vi "rad_Deploy Image Wrapper_FB.vi"(4 "Deploy":string[](array[string]), 6 "restart after imaging (T)":bool=TRUE, 7 "Deployment Notifiers":T3, 8 "error in (no error)":errorcluster, 9 "apply primary NIC from image (F)":bool, 10 "image file path":path, 11 "Target settings in":T1={"Hostname"="", "Serial number"="", "Product name"="", "Product code"=0, "System status"="", "Credential type"=enum."None/Unlocked", "User added?"=FALSE, "Primary NIC"={"MAC address"="", "IP Address Request Mode"=2, "IP address"="", "Subnet mask"="", "Gateway"="", "DNS server"=""}} {"Primary NIC"."IP Address Request Mode" items=["Static"=1, "DHCP/Link-Local"=2, "Link-Local Only"=4, "DHCP Only"=8]}) -> (0 "error out":errorcluster, 2 "image file path":path, 3 "Target settings out":T1={"Hostname"="", "Serial number"="", "Product name"="", "Product code"=0, "System status"="", "Credential type"=enum."None/Unlocked", "User added?"=FALSE, "Primary NIC"={"MAC address"="", "IP Address Request Mode"=2, "IP address"="", "Subnet mask"="", "Gateway"="", "DNS server"=""}} {"Primary NIC"."IP Address Request Mode" items=["Static"=1, "DHCP/Link-Local"=2, "Link-Local Only"=4, "DHCP Only"=8]})   [LabVIEW 2016]
uses:
  TypeDefs/rad_Deployment Notifiers.ctl
  TypeDefs/rad_Deployment Status Data Type.ctl
  TypeDefs/rad_Deployment Progress Data Type.ctl
  Targets/TypeDefs/rad_Target Information.ctl
  Targets/TypeDefs/rad_Target Network Settings.ctl
  <vilib>/nisyscfg/Network Settings Image.ctl
  <vilib>/nisyscfg/Set System Image (Folder).vi
  <vilib>/nisyscfg/Close (System).vi
  <vilib>/nisyscfg/nisyscfg.lvlib
panel:
  out "Product name":string
  out "finished":bool
  in  "Stop Checking for Events":bool
  out "Progress":u8(slide) scale=0.0..100.0
  out "Status":string
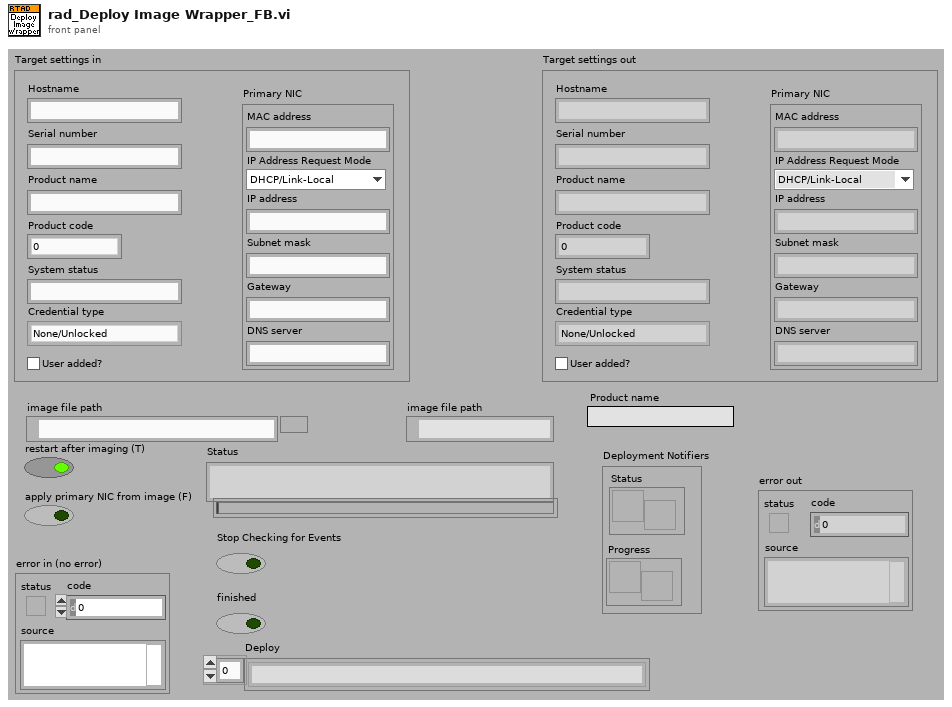
[diagram p1: front panel]
types:
  T1 = typedef "rad_Target Information.ctl" = cluster{"Hostname":string, "Serial number":string, "Product name":string, "Product code":i32, "System status":string, "Credential type":enum16{"None/Unlocked", "FTP Password", "NIAuth Credentials"}, "User added?":bool, "Primary NIC":T2}
  T2 = typedef "rad_Target Network Settings.ctl" = cluster{"MAC address":string, "IP Address Request Mode":i32, "IP address":string, "Subnet mask":string, "Gateway":string, "DNS server":string}
  T3 = typedef "rad_Deployment Notifiers.ctl" = cluster{"Status":refnum<notifier>, "Progress":refnum<notifier>}
  T4 = typedef "rad_Deployment Progress Data Type.ctl" = i8
  T5 = typedef "nisyscfg.lvlib/Network Settings Image.ctl" = u32
  T6 = enum32{"state changed", "beginning restart", "getting file", "putting file", "creating directory", "deleting file", "deleting directory", "enumerating file system", "renaming file", "current component", "operation progress", "downloading file", "unpacking file", "running install script"}
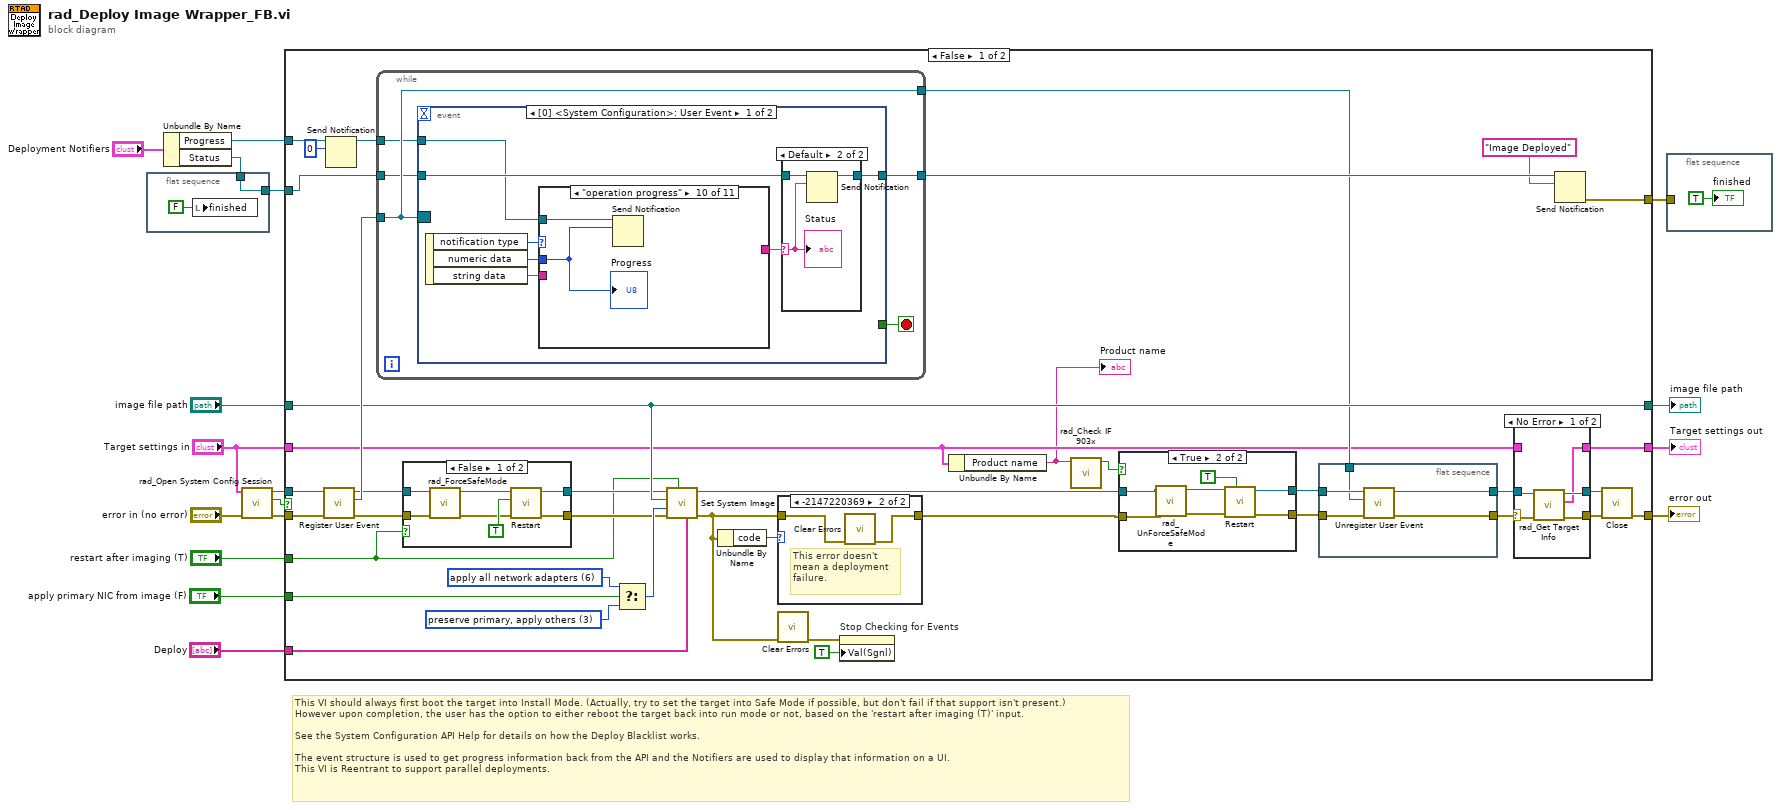
[diagram p0: block diagram]
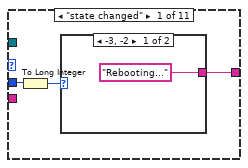
[diagram p7: hidden frame]
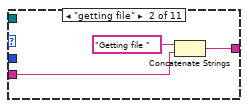
[diagram p9: hidden frame]
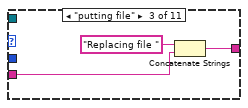
[diagram p10: hidden frame]
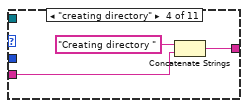
[diagram p11: hidden frame]
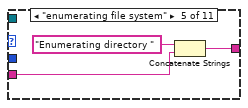
[diagram p12: hidden frame]
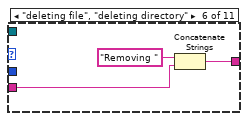
[diagram p13: hidden frame]
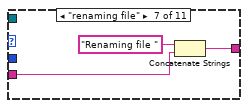
[diagram p14: hidden frame]
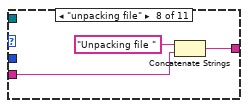
[diagram p15: hidden frame]
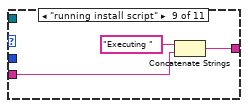
[diagram p16: hidden frame]
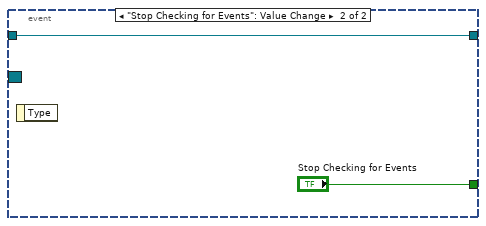
[diagram p18: hidden frame]
diagram:
  # "This VI should always first boot the target into Install Mode. (Actually, try to set the target into Safe Mode if possible, but don't fail if that support isn't present.)\nHowever upon completion, the user has the option to either reboot the target back into run mode or not, based on the 'restart after imaging (T)' input.\n\nSee the System Configuration API Help for details on how the Deploy Blacklist works.\n\nThe event structure is used to get progress information back from the API and the Notifiers are used to display that information on a UI. \nThis VI is Reentrant to support parallel deployments."
  n1 = flat-sequence {
    tunnel: [w18] -> w3
    tunnel: w2 -> [w18]
    frame #0 {
      n2 = local write "finished"(FALSE ("finished")) -> ()
    }
  }
  n3 = Unbundle By Name("Deployment Notifiers") -> ("Progress"=w11:refnum<notifier>, "Status"=w2:refnum<notifier>)
  n4 = call "rad_Open System Config Session.vi"("error in (no error)"="error in (no error)", "Target settings"="Target settings in") -> ("error out"=w7:errorcluster, "Cancelled"=w6:bool, "Session out"=w8:refnum<k21>)  [unwired: 6 in, 1 out]
  n5 = case shown="False" w6 {
    tunnel: [w58 w143] -> w17
    tunnel: "image file path" -> [w44 w142]
    tunnel: "restart after imaging (T)" -> [w37 _]
    tunnel: w8 -> [w57 _]
    tunnel: w7 -> [w56 w143]
    tunnel: [w52 _] -> w14
    tunnel: "apply primary NIC from image (F)" -> [w51 _]
    tunnel: w11 -> [w47 _]
    tunnel: [w44 w142] -> w16
    tunnel: "Deploy" -> [w43 _]
    tunnel: "Target settings in" -> [w26 w141]
    tunnel: [w34 w141] -> w4
    tunnel: w3 -> [w30 _]
    frame False {
      w50 = T5 6 items=["reset primary, disable others", "preserve primary, disable others", "preserve all network adapters", "preserve primary, apply others", "apply primary, disable others", "apply primary, preserve others", "apply all network adapters"] ("network settings (apply all adapters)")
      w49 = T5 3 items=["reset primary, disable others", "preserve primary, disable others", "preserve all network adapters", "preserve primary, apply others", "apply primary, disable others", "apply primary, preserve others", "apply all network adapters"] ("network settings (apply all adapters)")
      n6 = call <vilib>:"Register User Event.vi"("error in (no error)"=w56, "Session in"=w57) -> ("error out"=w40:errorcluster, "Event Registration out"=w55:refnum<event-registration>, "Session out"=w41:refnum<k21>)  [unwired: 7 in]
      n7 = Send Notification(notification=T4 0, notifier=w47) -> (notifier out=w46:refnum<notifier>)  [unwired: 1 in, 1 out]
      n8 = while {
        tunnel: w55 -> [w97]
        tunnel: [w97] -> w33
        tunnel: w30 -> [w95]
        tunnel: [w94] -> w54
        tunnel: w46 -> [w93]
        stop <- w96 stop-if-true
        n9 = event shown="[0] <System Configuration>: User Event" {
          selector: w97 -> [_ _]
          dyn-events: _ -> [_ _]
          timeout: _ -> [_ _]
          tunnel: [_ "Stop Checking for Events"] -> w96
          tunnel: w95 -> [w100 w139]
          tunnel: [w99 w139] -> w94
          tunnel: w93 -> [w98 _]
          event User Event {
            n10 = event-data() -> ("notification type"=w104:T6, "numeric data"=w102:u32, "string data"=w103:string)  [unwired: 1 in]
            n11 = case shown="\"operation progress\"" w104 {
              tunnel: [w109 w113 w116 w119 w122 w125 w128 w131 w134 _ _] -> w101
              tunnel: w103 -> [_ w114 w117 w120 w123 w126 w129 w132 w135 _ _]
              tunnel: w102 -> [w111 _ _ _ _ _ _ _ _ w138 _]
              tunnel: w98 -> [_ _ _ _ _ _ _ _ _ w137 _]
              frame "state changed" {
                n12 = To Long Integer(number=w111) -> (32bit integer=w110:i32)
                n13 = case shown="-3, -2" w110 {
                  tunnel: ["Rebooting..." _] -> w109
                  frame -3, -2 {
                  }
                  frame Default {
                  }
                }
              }
              frame "getting file" {
                n14 = Concatenate Strings("Getting file " ("Status"), w114) -> (w113:string)
              }
              frame "putting file" {
                n15 = Concatenate Strings("Replacing file " ("Status"), w117) -> (w116:string)
              }
              frame "creating directory" {
                n16 = Concatenate Strings("Creating directory " ("Status"), w120) -> (w119:string)
              }
              frame "enumerating file system" {
                n17 = Concatenate Strings("Enumerating directory " ("Status"), w123) -> (w122:string)
              }
              frame "deleting file", "deleting directory" {
                n18 = Concatenate Strings("Removing " ("Status"), w126) -> (w125:string)
              }
              frame "renaming file" {
                n19 = Concatenate Strings("Renaming file " ("Status"), w129) -> (w128:string)
              }
              frame "unpacking file" {
                n20 = Concatenate Strings("Unpacking file " ("Status"), w132) -> (w131:string)
              }
              frame "running install script" {
                n21 = Concatenate Strings("Executing " ("Status"), w135) -> (w134:string)
              }
              frame "operation progress" {
                n22 = Send Notification(notification=w138, notifier=w137) -> ()  [unwired: 1 in, 2 out]
                "Progress" <- w138
              }
              frame Default {
              }
            }
            n23 = case shown="Default" w101 {
              selector: w101 -> [_ w107]
              tunnel: w100 -> [w105 w108]
              tunnel: [w105 w106] -> w99
              frame "" {
              }
              frame Default {
                n24 = Send Notification(notification=w107, notifier=w108) -> (notifier out=w106:refnum<notifier>)  [unwired: 1 in, 1 out]
                "Status" <- w107
              }
            }
          }
          event "Stop Checking for Events": Value Change {
            n25 = event-data() -> ()  [unwired: 1 in, 1 out]
          }
        }
      }
      n26 = case shown="False" w37 {
        tunnel: w41 -> [w82 w84]
        tunnel: w40 -> [w77 w83]
        tunnel: [w80 w84] -> w39
        tunnel: [w79 w83] -> w38
        frame False {
          n27 = call "rad_ForceSafeMode.vi"("error in (no error)"=w77, "Target in"=w82) -> ("error out"=w76:errorcluster, "Target out"=w78:refnum<k21>)  [unwired: 8 in]
          n28 = call <vilib>:"Restart.vi"("error in (no error)"=w76, "Install Mode (F)"=TRUE ("install mode (F)"), "Session in"=w78) -> ("error out"=w79:errorcluster, "Session out"=w80:refnum<k21>)  [unwired: 6 in, 1 out]
        }
        frame True {
        }
      }
      n29 = Select(t=w50, s=w51, f=w49) -> (s? t:f=w48:T5)
      n30 = call-poly <vilib>:"Set System Image.vi"("File and Directory Blacklist"=w43, "Restart Automatically (T)"=w37, "error in (no error)"=w38, "Network Settings (preserve primary adapter, apply others)"=w48, "Source Folder"=w44, "Session in"=w39) -> ("error out"=w28:errorcluster, "Session out"=w23:refnum<k21>)  [unwired: 4 in]
      n31 = Unbundle By Name(w28) -> ("code"=w42:i32)
      n32 = case shown="-2147220369" w42 {
        tunnel: w28 -> [w85 w87]
        tunnel: [w85 w86] -> w22
        frame Default {
        }
        frame -2147220369 {
          # "This error doesn't\nmean a deployment\nfailure."
          n33 = call <vilib>:"Clear Errors.vi"("error in (no error)"=w87) -> ("error out"=w86:errorcluster)  [unwired: 5 in, 1 out]
        }
      }
      n34 = call <vilib>:"Clear Errors.vi"("error in (no error)"=w28) -> ("error out"=w27:errorcluster)  [unwired: 5 in, 1 out]
      n35 = property on="Stop Checking for Events" class="Bool (strict)"(error in=w27, "Val(Sgnl)"=TRUE ("Stop Checking for Events")) -> ()  [unwired: 1 in, 2 out]
      n36 = Unbundle By Name(w26) -> ("Product name"=w25:string)
      "Product name" <- w25
      n37 = call "rad_Check IF 903x.vi"("Product Name"=w25) -> ("Found 903x?"=w24:bool)  [unwired: 10 in]
      n38 = case shown="True" w24 {
        tunnel: w23 -> [w60 w67]
        tunnel: w22 -> [w59 w66]
        tunnel: [w59 w63] -> w21
        tunnel: [w60 w62] -> w20
        frame False {
        }
        frame True {
          n39 = call "rad_UnForceSafeMode.vi"("error in (no error)"=w66, "Target in"=w67) -> ("error out"=w64:errorcluster, "Target out"=w65:refnum<k21>)  [unwired: 8 in]
          n40 = call <vilib>:"Restart.vi"("Wait Until Complete (T)"=TRUE, "error in (no error)"=w64, "Session in"=w65) -> ("error out"=w63:errorcluster, "Session out"=w62:refnum<k21>)  [unwired: 6 in, 1 out]
        }
      }
      n41 = flat-sequence {
        tunnel: w21 -> [w92]
        tunnel: w20 -> [w91]
        tunnel: w33 -> [w90]
        tunnel: [w89] -> w32
        tunnel: [w88] -> w31
        frame #0 {
          n42 = call <vilib>:"Unregister User Event.vi"("error in (no error)"=w92, "Event Registration in"=w90, "Session in"=w91) -> ("error out"=w89:errorcluster, "Session out"=w88:refnum<k21>)  [unwired: 7 in]
        }
      }
      n43 = case shown="No Error" w32 {
        selector: w32 -> [w71 w75]
        tunnel: [w69 w75] -> w36
        tunnel: w31 -> [w72 w74]
        tunnel: [w70 w74] -> w35
        tunnel: [w68 w73] -> w34
        tunnel: w26 -> [_ w73]
        frame No Error {
          n44 = call "rad_Get Target Info.vi"("error in (no error)"=w71, "System Session in"=w72) -> ("error out"=w69:errorcluster, "Target settings"=w68:T1, "System Session out"=w70:refnum<k21>)  [unwired: 7 in]
        }
        frame Error {
        }
      }
      n45 = Send Notification(notification="Image Deployed", notifier=w54) -> (error out=w52:errorcluster)  [unwired: 1 in, 1 out]
      n46 = call-poly <vilib>:"Close.vi"("error in (no error)"=w36, "Session in"=w35) -> ("error out"=w58:errorcluster)  [unwired: 9 in]
    }
    frame True {
    }
  }
  "error out" <- w17
  "image file path" <- w16
  "Target settings out" <- w4
  n47 = flat-sequence {
    tunnel: w14 -> [_]
    frame #0 {
      "finished" <- TRUE ("finished")
    }
  }
